vi "Write gnd time.vi"(8 "error in (no error)":errorcluster caption="에러 입력(에러 없음)", 10 "gnd time":u8=3, 11 "Auto Tracking Wave 입력":refnum<class "Auto Track Wave.lvclass">) -> (0 "error out":errorcluster caption="에러 출력", 3 "Auto Tracking Wave 출력":refnum<class "Auto Track Wave.lvclass">)   [LabVIEW 2020, in "Auto Track Wave.lvclass"]
uses:
  Auto Track Wave.lvclass
  Auto Track Wave.lvclass/Auto Track Wave.ctl
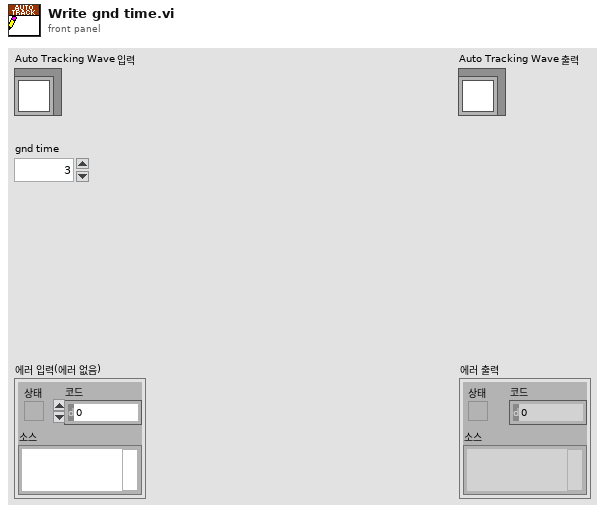
[diagram p1: front panel]
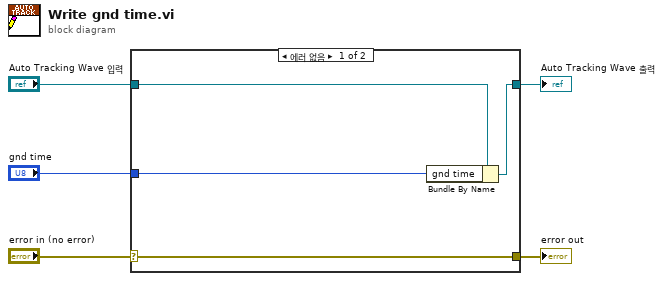
[diagram p0: block diagram]
diagram:
  n1 = case shown="에러 없음" "error in (no error)" {
    selector: "error in (no error)" -> [w9 w10]
    tunnel: [w9 w10] -> w4
    tunnel: [w7 w11] -> w2
    tunnel: "Auto Tracking Wave 입력" -> [w8 w11]
    tunnel: "gnd time" -> [w6 _]
    frame No Error {
      n2 = Bundle By Name(cluster=w8, "gnd time"=w6) -> (w7:refnum<class "Auto Track Wave.lvclass">)
    }
    frame Error {
    }
  }
  "error out" <- w4
  "Auto Tracking Wave 출력" <- w2
